vi "svl_Limit Testing (array) (scalar limits).vi"(9 "lower limit":dbl format="%.2f", 10 "input array":dbl[](array[numeric]) format="%.2f", 11 "upper limit":dbl format="%.2f") -> (1 "lower limit array":dbl[](array[numeric]) format="%.2f", 2 "failure array":dbl[](array[numeric]) format="%.2f", 3 "upper limit array":dbl[](array[numeric]) format="%.2f", 4 "test passed":bool, 6 "test results":bool[](array[boolean]))   [LabVIEW 2017, in "SoundVib_LimitTest.lvlib"]
uses:
  <vilib>/addons/Sound and Vibration/svt_Limit Test/SoundVib_LimitTest.lvlib
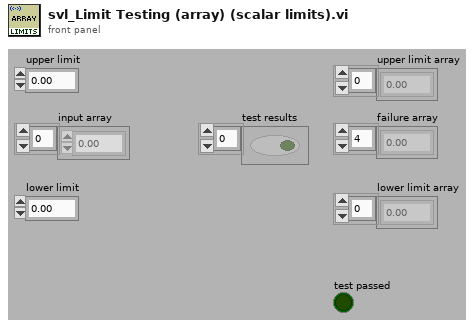
[diagram p1: front panel]
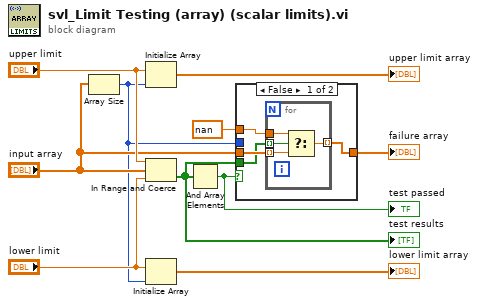
[diagram p0: block diagram]
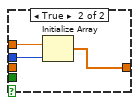
[diagram p2: hidden frame]
diagram:
  n1 = Array Size(array="input array") -> (size(s)=w1:i32)
  n2 = Initialize Array("upper limit", w1) -> (→"upper limit array":dbl[])
  n3 = In Range and Coerce(upper limit="upper limit", x="input array", lower limit="lower limit") -> (In Range?=w10:bool[])  [unwired: 1 out]
  "test results" <- w10
  n4 = Initialize Array("lower limit", w1) -> (→"lower limit array":dbl[])
  n5 = And Array Elements(Boolean array=w10) -> (logical AND=w3:bool)
  "test passed" <- w3
  n6 = case shown="False" w3 {
    tunnel: w10 -> [w13 _]
    tunnel: "input array" -> [w14 _]
    tunnel: [w12 w19] -> w9
    tunnel: nan ("element") -> [w11 w21]
    tunnel: w1 -> [_ w20]
    frame False {
      n7 = for {
        tunnel: w14 -> [w16] mode=indexing
        tunnel: w13 -> [w18] mode=indexing
        tunnel: w11 -> [w15]
        tunnel: [w17] -> w12 mode=indexing
        n8 = Select(t=w15, s=w18, f=w16) -> (s? t:f=w17:dbl)
      }
    }
    frame True {
      n9 = Initialize Array(w21, w20) -> (w19:dbl[])
    }
  }
  "failure array" <- w9
